vi "General Polynomial Fit PtByPt.vi"(4 "sample length":i32=100, 5 "initialize":bool, 6 "algorithm":T1(ring), 7 "polynomial order":i32=2, 8 "x":dbl format="%0.2f", 9 "y":dbl format="%0.2f") -> (0 "error":i32, 1 "mse":dbl format="%0.2f", 2 "Polynomial Fit Coefficients":dbl[](array[numeric]), 3 "Best Polynomial Fit":dbl[](array[numeric]))   [LabVIEW 2020, in "NI_PtbyPt.lvlib"]
doc: "Finds the polynomial curve values and the set of <B>Polynomial Fit Coefficients</B> which describe the polynomial curve that best represents the set of input data points specified by <B>sample length</B>."
uses:
  <vilib>/ptbypt/NI_PtbyPt.lvlib
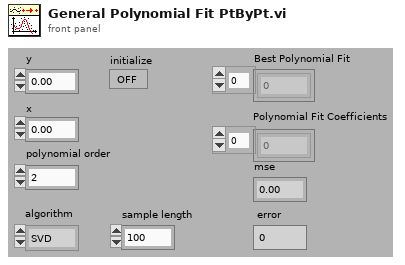
[diagram p1: front panel]
types:
  T1 = enum32{"SVD", "Givens", "Givens2", "Householder", "LU Decomposition", "Cholesky"}
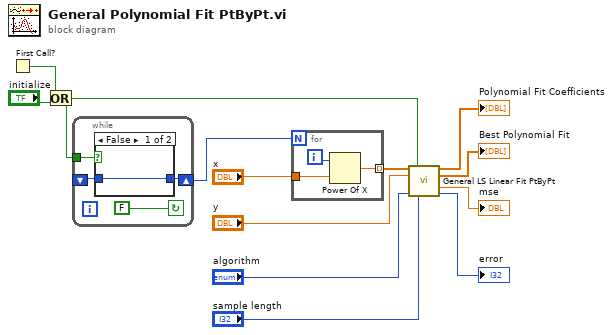
[diagram p0: block diagram]
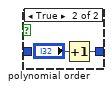
[diagram p2: hidden frame]
diagram:
  n1 = First Call?() -> (First Call?: T/F=w3:bool)
  n2 = Or(x=w3, y="initialize") -> (x .or. y?=w2:bool)
  n3 = while {
    shift-left: _ -> [w15]
    shift-right: [w16] -> w1
    tunnel: w2 -> [w17]
    stop <- FALSE continue-if-true
    n4 = case shown="False" w17 {
      tunnel: [w18 w19] -> w16
      tunnel: w15 -> [w18 _]
      frame False {
      }
      frame True {
        n5 = Increment(x="polynomial order") -> (x+1=w19:i32)
      }
    }
  }
  n6 = for {
    N: w1 -> [_]
    tunnel: [w22] -> w10 mode=indexing
    tunnel: "x" -> [w21]
    i -> [w23]
    n7 = Power Of X(1:w21, 2:w23) -> (0:w22:dbl)
  }
  n8 = call <vilib>:"General LS Linear Fit PtByPt.vi"("H"=w10, "initialize"=w2, "y"="y", "algorithm"="algorithm", "sample length"="sample length") -> ("Coefficients"=→"Polynomial Fit Coefficients":dbl[], "Best Fit"=→"Best Polynomial Fit":dbl[], "mse"=→"mse":dbl, "error"=→"error":i32)  [unwired: 6 in, 1 out]
